vi "WaterMixRatios2Calibrate.vi"(10 "Base Dilution":dbl, 11 "Mix Sequence Array":bool[][](array[boolean])) -> (2 "numOdor":i32[](array[numeric]), 3 "waterRatio":dbl[](array[numeric]))   [LabVIEW 2016]
uses:
  <vilib>/imath/engines/lvmath2/RunTimeEngine/BuiltInFunctions/size/NIMS_I32=size(GM,I32).vi
  <instcachedir>/0/NIMS_I32=size(GM,I32)_9B6975FE2A37478D9DF1A6A9597B9E6B.lvgen/NIMS_I32=size(GM,I32)_9B6975FE2A37478D9DF1A6A9597B9E6B_005.vi
  <vilib>/imathl/engines/lvmath/Functions/Error Handling/Create Error.vi
  <vilib>/imath/engines/lvmath2/RunTimeEngine/RangeToken/NIMS_Range_R2 - Integer.vi
  <instcachedir>/0/NIMS_Range_R2 - Integer_416A044C4F024DBE8E97DA138CB3186F.lvgen/NIMS_Range_R2 - Integer_416A044C4F024DBE8E97DA138CB3186F_000.vi
  <vilib>/imath/engines/lvmath2/RunTimeEngine/CommandStatement/MC_CommandStatement_break.vi
  <vilib>/imath/engines/lvmath2/RunTimeEngine/VariableToken/NIMS_VariableToken_CondDefinedDefinedByReplace.vi
  <instcachedir>/0/NIMS_VariableToken_CondDefinedDefinedByReplace_D162CFFC24174562A9FEA619A91E1A56.lvgen/NIMS_VariableToken_CondDefinedDefinedByReplace_D162CFFC24174562A9FEA619A91E1A56_004.vi
  <vilib>/imath/engines/lvmath2/RunTimeEngine/IndexRead/NIMS M(S,$).vi
  <instcachedir>/0/NIMS M(S,$)_F24F360562DE41D8BE234322A2E15C65.lvgen/NIMS M(S,$)_F24F360562DE41D8BE234322A2E15C65_002.vi
  <vilib>/imath/engines/lvmath2/RunTimeEngine/BuiltInFunctions/findnz/NIMS_[1o]_findnz(GRowV).vi
  <instcachedir>/0/NIMS_[1o]_findnz(GRowV)_656056C849EF4762B1F0843BDDDEF2FF.lvgen/NIMS_[1o]_findnz(GRowV)_656056C849EF4762B1F0843BDDDEF2FF_000.vi
  <vilib>/imath/engines/lvmath2/RunTimeEngine/BuiltInFunctions/length/NIMS_length(GV).vi
  <instcachedir>/0/NIMS_length(GV)_08A3D13377FD4E4B96F5795FBF3698FA.lvgen/NIMS_length(GV)_08A3D13377FD4E4B96F5795FBF3698FA_002.vi
  <vilib>/imath/engines/lvmath2/RunTimeEngine/IndexReplace/NIMS V(S)=S.vi
  <instcachedir>/0/NIMS V(S)=S_5B9D821375184D3582A2146CD1A04ED7.lvgen/NIMS V(S)=S_5B9D821375184D3582A2146CD1A04ED7_003.vi
  <vilib>/imath/engines/lvmath2/RunTimeEngine/ErrorHandling/NIMS_Create Error From Enums.vi
  <vilib>/imath/engines/lvmath2/RunTimeEngine/VariableToken/NIMS_VariableToken_CondDefined.vi
  <instcachedir>/0/NIMS_VariableToken_CondDefined_620A15720FCC4DA7863546285C12295E.lvgen/NIMS_VariableToken_CondDefined_620A15720FCC4DA7863546285C12295E_005.vi
  <vilib>/imath/engines/lvmath2/RunTimeEngine/BuiltInFunctions/sets_unique/NIMS_sets_unique(GV).vi
  <instcachedir>/0/NIMS_sets_unique(GV)_BC60CBD939E647F382369330BF9EA64D.lvgen/NIMS_sets_unique(GV)_BC60CBD939E647F382369330BF9EA64D_007.vi
  <vilib>/imath/engines/lvmath2/RunTimeEngine/NodeEndStatement/NIMS_NodeEndStatement_Output.vi
  <instcachedir>/0/NIMS_NodeEndStatement_Output_53EC0D466D134D7ABD903AC30B43404B.lvgen/NIMS_NodeEndStatement_Output_53EC0D466D134D7ABD903AC30B43404B_005.vi
  <instcachedir>/0/NIMS_NodeEndStatement_Output_53EC0D466D134D7ABD903AC30B43404B.lvgen/NIMS_NodeEndStatement_Output_53EC0D466D134D7ABD903AC30B43404B_004.vi
  <vilib>/imath/engines/lvmath2/RunTimeEngine/ErrorHandling/NIMS_Finalize Error.vi
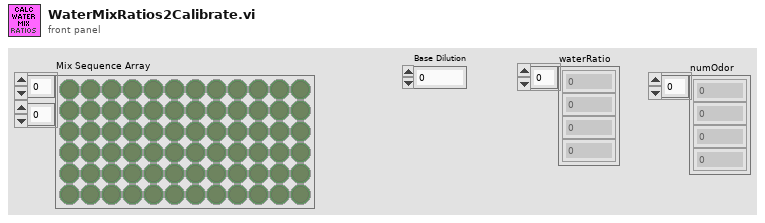
[diagram p1: front panel]
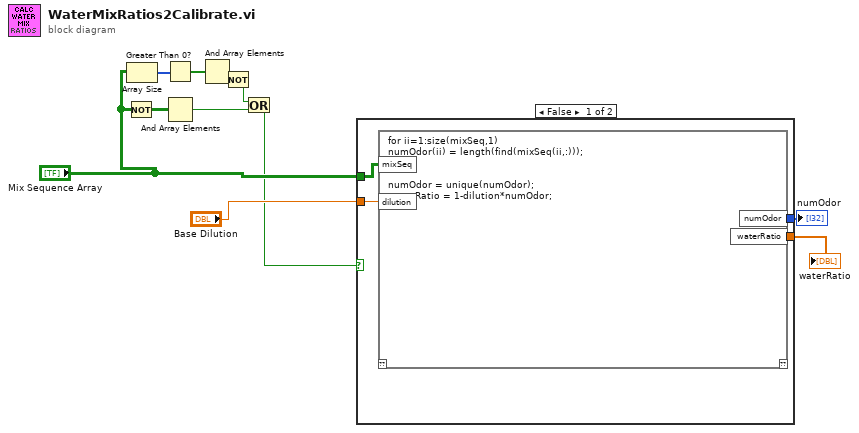
[diagram p0: block diagram]
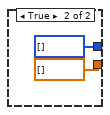
[diagram p2: hidden frame]
diagram:
  n1 = Not(x="Mix Sequence Array") -> (.not. x?=w6:bool[][])
  n2 = Array Size(array="Mix Sequence Array") -> (size(s)=w8:i32[])
  n3 = Greater Than 0?(x=w8) -> (x > 0?=w7:bool[])
  n4 = And Array Elements(Boolean array=w6) -> (logical AND=w4:bool)
  n5 = And Array Elements(Boolean array=w7) -> (logical AND=w5:bool)
  n6 = Not(x=w5) -> (.not. x?=w3:bool)
  n7 = Or(x=w3, y=w4) -> (x .or. y?=w1:bool)
  n8 = case shown="False" w1 {
    tunnel: "Base Dilution" -> [w15 _]
    tunnel: [w14 i32[] [] ("numOdor")] -> w10
    tunnel: [w13 dbl[] [] ("waterRatio")] -> w9
    tunnel: "Mix Sequence Array" -> [w12 _]
    frame False {
      n9 = mathscript code="for ii=1:size(mixSeq,1)\nnumOdor(ii) = length(find(mixSeq(ii,:)));\nend\n\nnumOdor = unique(numOdor);\nwaterRatio = 1-dilution*numOdor;"("mixSeq"=w12, "dilution"=w15) -> ("numOdor"=w14:i32[], "waterRatio"=w13:dbl[])  [unwired: 1 in, 1 out]
    }
    frame True {
    }
  }
  "numOdor" <- w10
  "waterRatio" <- w9
